vi "输入数据解析.vi"(0 "单个参数补充":dbl, 1 "从板号":dbl=1.0, 2 "主板二维码":string="BNET01", 3 "从板二维码":string="BNET01", 5 "主板引用":refnum<vi>, 7 "从板引用":refnum<vi>, 9 "主板选项":string="三级故障阀值", 11 "枚举":enum16{"主板", "从板"}(ring), 12 "快换":bool caption="快换写入") -> (4 "输出数组":dbl[][](array[numeric]), 6 "数组长度":dbl[](array[numeric]), 8 "循环次数":i32, 10 "命令":u32, 14 "名称":string[](array[string]), 15 "命令序号":u32[](array[numeric]))   [LabVIEW 2013] (continued)
                  }
                  frame Enabled {
                    w11585 = 255 ("高字节1")
                  }
                }
                n4442 = Build Array(w11577, w11578) -> (w11576:i32[])
              }
              frame 2 {
                # "温度过高"
                n4443 = disable-structure shown="启用" {
                  disable-tunnel: [w11592 255 ("高字节1")] -> w11588
                  disable-tunnel: w11586 -> [w11590 _]
                  frame Disabled {
                    n4444 = Unbundle By Name(w11590) -> ("温度过高"=w11589:dbl)
                    n4445 = call "输入分辨率计算-EV05.vi"("1字节?"=TRUE, "数值"=w11589, "偏移量"=-40.0, "分辨率"=1.0) -> ("高字节1"=w11592:dbl)  [unwired: 1 in, 6 out]
                  }
                  frame Enabled {
                  }
                }
                n4446 = Build Array(w11588) -> (w11587:i32[])
              }
              frame 3 {
                # "温度过低"
                n4447 = disable-structure shown="启用" {
                  disable-tunnel: [w11602 255 ("高字节1")] -> w11598
                  disable-tunnel: w11596 -> [w11600 _]
                  frame Disabled {
                    n4448 = Unbundle By Name(w11600) -> ("温度过低"=w11599:dbl)
                    n4449 = call "输入分辨率计算-EV05.vi"("1字节?"=TRUE, "数值"=w11599, "偏移量"=-40.0, "分辨率"=1.0) -> ("高字节1"=w11602:dbl)  [unwired: 1 in, 6 out]
                  }
                  frame Enabled {
                  }
                }
                n4450 = Build Array(w11598) -> (w11597:i32[])
              }
              frame 4 {
                # "整组温度不均衡"
                n4451 = disable-structure shown="启用" {
                  disable-tunnel: [w11612 255 ("高字节1")] -> w11608
                  disable-tunnel: w11606 -> [w11610 _]
                  frame Disabled {
                    n4452 = Unbundle By Name(w11610) -> ("整组温度不均衡"=w11609:dbl)
                    n4453 = call "输入分辨率计算-EV05.vi"("1字节?"=TRUE, "数值"=w11609, "偏移量"=0.0, "分辨率"=1.0) -> ("高字节1"=w11612:dbl)  [unwired: 1 in, 6 out]
                  }
                  frame Enabled {
                  }
                }
                n4454 = Build Array(w11608) -> (w11607:i32[])
              }
              frame 5 {
                # "单组电压不均衡"
                n4455 = disable-structure shown="启用" {
                  disable-tunnel: [w11624 w11627] -> w11619
                  disable-tunnel: [w11622 w11627] -> w11617
                  disable-tunnel: w11616 -> [w11621 _]
                  frame Disabled {
                    n4456 = Unbundle By Name(w11621) -> ("单组电压不均衡"=w11620:dbl)
                    n4457 = call "输入分辨率计算-EV05.vi"("1字节?"=FALSE, "数值"=w11620, "偏移量"=0.0, "分辨率"=0.001) -> ("低字节"=w11622:dbl, "高字节1"=w11624:dbl)  [unwired: 1 in, 5 out]
                  }
                  frame Enabled {
                    w11627 = 255 ("高字节1")
                  }
                }
                n4458 = Build Array(w11619, w11617) -> (w11618:i32[])
              }
              frame 6 {
                # "整组电压不均衡"
                n4459 = disable-structure shown="启用" {
                  disable-tunnel: [w11636 w11639] -> w11631
                  disable-tunnel: [w11634 w11639] -> w11629
                  disable-tunnel: w11628 -> [w11633 _]
                  frame Disabled {
                    n4460 = Unbundle By Name(w11633) -> ("整组电压不均衡"=w11632:dbl)
                    n4461 = call "输入分辨率计算-EV05.vi"("1字节?"=FALSE, "数值"=w11632, "偏移量"=0.0, "分辨率"=0.001) -> ("低字节"=w11634:dbl, "高字节1"=w11636:dbl)  [unwired: 1 in, 5 out]
                  }
                  frame Enabled {
                    w11639 = 255 ("高字节1")
                  }
                }
                n4462 = Build Array(w11631, w11629) -> (w11630:i32[])
              }
              frame 7 {
                # "单体电压过高"
                n4463 = disable-structure shown="启用" {
                  disable-tunnel: [w11648 w11651] -> w11643
                  disable-tunnel: [w11646 w11651] -> w11641
                  disable-tunnel: w11640 -> [w11645 _]
                  frame Disabled {
                    n4464 = Unbundle By Name(w11645) -> ("单体电压过高"=w11644:dbl)
                    n4465 = call "输入分辨率计算-EV05.vi"("1字节?"=FALSE, "数值"=w11644, "偏移量"=0.0, "分辨率"=0.001) -> ("低字节"=w11646:dbl, "高字节1"=w11648:dbl)  [unwired: 1 in, 5 out]
                  }
                  frame Enabled {
                    w11651 = 255 ("高字节1")
                  }
                }
                n4466 = Build Array(w11643, w11641) -> (w11642:i32[])
              }
              frame 8 {
                # "单体电压过低"
                n4467 = disable-structure shown="启用" {
                  disable-tunnel: [w11660 w11663] -> w11655
                  disable-tunnel: [w11658 w11663] -> w11653
                  disable-tunnel: w11652 -> [w11657 _]
                  frame Disabled {
                    n4468 = Unbundle By Name(w11657) -> ("单体电压过低"=w11656:dbl)
                    n4469 = call "输入分辨率计算-EV05.vi"("1字节?"=FALSE, "数值"=w11656, "偏移量"=0.0, "分辨率"=0.001) -> ("低字节"=w11658:dbl, "高字节1"=w11660:dbl)  [unwired: 1 in, 5 out]
                  }
                  frame Enabled {
                    w11663 = 255 ("高字节1")
                  }
                }
                n4470 = Build Array(w11655, w11653) -> (w11654:i32[])
              }
              frame 9 {
                # "充电电流过高"
                n4471 = disable-structure shown="启用" {
                  disable-tunnel: [w11672 w11675] -> w11667
                  disable-tunnel: [w11670 w11675] -> w11665
                  disable-tunnel: w11664 -> [w11669 _]
                  frame Disabled {
                    n4472 = Unbundle By Name(w11669) -> ("充电电流过高"=w11668:dbl)
                    n4473 = call "输入分辨率计算-EV05.vi"("1字节?"=FALSE, "数值"=w11668, "偏移量"=-3000.0, "分辨率"=0.1) -> ("低字节"=w11670:dbl, "高字节1"=w11672:dbl)  [unwired: 1 in, 5 out]
                  }
                  frame Enabled {
                    w11675 = 255 ("高字节1")
                  }
                }
                n4474 = Build Array(w11667, w11665) -> (w11666:i32[])
              }
              frame 10 {
                # "放电电流过高"
                n4475 = disable-structure shown="启用" {
                  disable-tunnel: [w11684 w11687] -> w11679
                  disable-tunnel: [w11682 w11687] -> w11677
                  disable-tunnel: w11676 -> [w11681 _]
                  frame Disabled {
                    n4476 = Unbundle By Name(w11681) -> ("放电电流过高"=w11680:dbl)
                    n4477 = call "输入分辨率计算-EV05.vi"("1字节?"=FALSE, "数值"=w11680, "偏移量"=-3000.0, "分辨率"=0.1) -> ("低字节"=w11682:dbl, "高字节1"=w11684:dbl)  [unwired: 1 in, 5 out]
                  }
                  frame Enabled {
                    w11687 = 255 ("高字节1")
                  }
                }
                n4478 = Build Array(w11679, w11677) -> (w11678:i32[])
              }
              frame 11 {
                # "单组温度不均衡"
                n4479 = disable-structure shown="启用" {
                  disable-tunnel: [w11694 255 ("高字节1")] -> w11690
                  disable-tunnel: w11688 -> [w11692 _]
                  frame Disabled {
                    n4480 = Unbundle By Name(w11692) -> ("单组温度不均衡"=w11691:dbl)
                    n4481 = call "输入分辨率计算-EV05.vi"("1字节?"=TRUE, "数值"=w11691, "偏移量"=0.0, "分辨率"=1.0) -> ("高字节1"=w11694:dbl)  [unwired: 1 in, 6 out]
                  }
                  frame Enabled {
                  }
                }
                n4482 = Build Array(w11690) -> (w11689:i32[])
              }
              frame 12 {
                # "SOC过高"
                n4483 = Unbundle By Name(w11701) -> ("SOC过高"=w11700:dbl)
                n4484 = call "输入分辨率计算-EV05.vi"("1字节?"=FALSE, "数值"=w11700, "偏移量"=0.0, "分辨率"=0.1) -> ("低字节"=w11698:dbl, "高字节1"=w11699:dbl)  [unwired: 1 in, 5 out]
                n4485 = Build Array(w11699, w11698) -> (w11703:dbl[])
              }
              frame 13 {
                # "SOC过低"
                n4486 = disable-structure shown="启用" {
                  disable-tunnel: w11708 -> [w11713 _]
                  disable-tunnel: [w11711 w11717] -> w11707
                  disable-tunnel: [w11710 w11717] -> w11706
                  frame Disabled {
                    n4487 = Unbundle By Name(w11713) -> ("SOC过低"=w11712:dbl)
                    n4488 = call "输入分辨率计算-EV05.vi"("1字节?"=FALSE, "数值"=w11712, "偏移量"=0.0, "分辨率"=0.1) -> ("低字节"=w11710:dbl, "高字节1"=w11711:dbl)  [unwired: 1 in, 5 out]
                  }
                  frame Enabled {
                    w11717 = 255 ("高字节1")
                  }
                }
                n4489 = Build Array(w11707, w11706) -> (w11709:i32[])
              }
              frame 14 {
                # "内阻过大"
                n4490 = disable-structure shown="启用" {
                  disable-tunnel: w11720 -> [w11725 _]
                  disable-tunnel: [w11721 255 ("高字节1")] -> w11718
                  frame Disabled {
                    n4491 = Unbundle By Name(w11725) -> ("内阻过大"=w11724:dbl)
                    n4492 = call "输入分辨率计算-EV05.vi"("1字节?"=TRUE, "数值"=w11724, "分辨率"=0.1) -> ("高字节1"=w11721:dbl)  [unwired: 2 in, 6 out]
                  }
                  frame Enabled {
                  }
                }
                n4493 = Build Array(w11718) -> (w11719:i32[])
              }
              frame 15 {
                # "极柱温度过高"
                n4494 = disable-structure shown="启用" {
                  disable-tunnel: w11729 -> [w11735 _]
                  disable-tunnel: [w11731 255 ("高字节1")] -> w11727
                  frame Disabled {
                    n4495 = Unbundle By Name(w11735) -> ("极柱温度过高"=w11734:dbl)
                    n4496 = call "输入分辨率计算-EV05.vi"("1字节?"=TRUE, "数值"=w11734, "偏移量"=-40.0, "分辨率"=1.0) -> ("高字节1"=w11731:dbl)  [unwired: 1 in, 6 out]
                  }
                  frame Enabled {
                  }
                }
                n4497 = Build Array(w11727) -> (w11728:i32[])
              }
              frame 16 {
                # "SOH过低"
                n4498 = disable-structure shown="启用" {
                  disable-tunnel: [w11752 w11760] -> w11739
                  disable-tunnel: w11738 -> [w11749 _]
                  disable-tunnel: [w11741 w11760] -> w11737
                  frame Disabled {
                    n4499 = Unbundle By Name(w11749) -> ("SOH过低"=w11748:dbl)
                    n4500 = call "输入分辨率计算-EV05.vi"("1字节?"=FALSE, "数值"=w11748, "偏移量"=0.0, "分辨率"=0.1) -> ("低字节"=w11750:dbl, "高字节1"=w11751:dbl)  [unwired: 1 in, 5 out]
                    n4501 = call "二进制解析-8.6.vi"("索引"=4, "数值"=w11751) -> ("低位子数组"=w11754:i32[])  [unwired: 3 out]
                    n4502 = call "二进制解析-8.6.vi"("索引"=4, "数值"=w11750) -> ("低位子数组"=w11743:i32[], "高位子数组"=w11753:i32[])  [unwired: 2 out]
                    n4503 = call "二进制解析-8.6.vi"("索引"=4, "数值"=0) -> ("低位子数组"=w11744:i32[])  [unwired: 3 out]
                    n4504 = Insert Into Array(array=w11754, new element=w11753) -> (w11747:i32[])  [unwired: 1 in]
                    n4505 = Insert Into Array(array=w11743, new element=w11744) -> (w11742:i32[])  [unwired: 1 in]
                    n4506 = call "数值二进制转十进制-8.6.vi"("子数组"=w11747) -> ("十进制数值"=w11752:i32)  [unwired: 4 out]
                    n4507 = call "数值二进制转十进制-8.6.vi"("子数组"=w11742) -> ("十进制数值"=w11741:i32)  [unwired: 4 out]
                  }
                  frame Enabled {
                    w11760 = 255 ("高字节1")
                  }
                }
                n4508 = Build Array(w11739, w11737) -> (w11740:i32[])
              }
            }
            n4509 = Insert Into Array(array=w11560, new element=w11561) -> (w11559:dbl[])  [unwired: 1 in]
          }
          n4510 = Build Array(w11556) -> (w11555:dbl[][])
          n4511 = Build Array("二级故障阀值") -> (w11546:string[])
        }
        frame "SOC过高(3)" {
          n4512 = Unbundle By Name(w11766) -> ("一级故障 3"=w11767:refnum<vi>)
          n4513 = property class="Clust (严格)"(reference=w11767) -> ("Value"=w11765:T4)  [unwired: 1 in, 2 out]
          n4514 = for {
            N: 17 -> [_]
            tunnel: w11765 -> [w11777]
            shift-right: [w11774] -> w11771
            shift-left: dbl[] [] -> [w11775]
            i -> [w11778]
            n4515 = case shown="12" w11778 {
              tunnel: w11777 -> [w11779 w11790 w11801 w11811 w11821 w11831 w11843 w11855 w11867 w11879 w11891 w11903 w11916 w11924 w11931 w11940 w11949]
              tunnel: [w11780 w11791 w11802 w11812 w11822 w11833 w11845 w11857 w11869 w11881 w11893 w11904 w11918 w11926 w11930 w11939 w11951] -> w11776
              frame 0, Default {
                # "总电压过高"
                n4516 = disable-structure shown="启用" {
                  disable-tunnel: [w11786 w11789] -> w11782
                  disable-tunnel: [w11785 w11789] -> w11781
                  disable-tunnel: w11779 -> [w11784 _]
                  frame Disabled {
                    n4517 = Unbundle By Name(w11784) -> ("总电压过高"=w11783:dbl)
                    n4518 = call "输入分辨率计算-EV05.vi"("1字节?"=FALSE, "数值"=w11783, "分辨率"=0.1) -> ("低字节"=w11786:dbl, "高字节1"=w11785:dbl)  [unwired: 2 in, 5 out]
                  }
                  frame Enabled {
                    w11789 = 255 ("高字节1")
                  }
                }
                n4519 = Build Array(w11781, w11782) -> (w11780:i32[])
              }
              frame 1 {
                # "总电压过低"
                n4520 = disable-structure shown="启用" {
                  disable-tunnel: [w11797 w11800] -> w11793
                  disable-tunnel: [w11796 w11800] -> w11792
                  disable-tunnel: w11790 -> [w11795 _]
                  frame Disabled {
                    n4521 = Unbundle By Name(w11795) -> ("总电压过低"=w11794:dbl)
                    n4522 = call "输入分辨率计算-EV05.vi"("1字节?"=FALSE, "数值"=w11794, "分辨率"=0.1) -> ("低字节"=w11797:dbl, "高字节1"=w11796:dbl)  [unwired: 2 in, 5 out]
                  }
                  frame Enabled {
                    w11800 = 255 ("高字节1")
                  }
                }
                n4523 = Build Array(w11792, w11793) -> (w11791:i32[])
              }
              frame 2 {
                # "温度过高"
                n4524 = disable-structure shown="启用" {
                  disable-tunnel: [w11807 255 ("高字节1")] -> w11803
                  disable-tunnel: w11801 -> [w11805 _]
                  frame Disabled {
                    n4525 = Unbundle By Name(w11805) -> ("温度过高"=w11804:dbl)
                    n4526 = call "输入分辨率计算-EV05.vi"("1字节?"=TRUE, "数值"=w11804, "偏移量"=-40.0, "分辨率"=1.0) -> ("高字节1"=w11807:dbl)  [unwired: 1 in, 6 out]
                  }
                  frame Enabled {
                  }
                }
                n4527 = Build Array(w11803) -> (w11802:i32[])
              }
              frame 3 {
                # "温度过低"
                n4528 = disable-structure shown="启用" {
                  disable-tunnel: [w11817 255 ("高字节1")] -> w11813
                  disable-tunnel: w11811 -> [w11815 _]
                  frame Disabled {
                    n4529 = Unbundle By Name(w11815) -> ("温度过低"=w11814:dbl)
                    n4530 = call "输入分辨率计算-EV05.vi"("1字节?"=TRUE, "数值"=w11814, "偏移量"=-40.0, "分辨率"=1.0) -> ("高字节1"=w11817:dbl)  [unwired: 1 in, 6 out]
                  }
                  frame Enabled {
                  }
                }
                n4531 = Build Array(w11813) -> (w11812:i32[])
              }
              frame 4 {
                # "整组温度不均衡"
                n4532 = disable-structure shown="启用" {
                  disable-tunnel: [w11827 255 ("高字节1")] -> w11823
                  disable-tunnel: w11821 -> [w11825 _]
                  frame Disabled {
                    n4533 = Unbundle By Name(w11825) -> ("整组温度不均衡"=w11824:dbl)
                    n4534 = call "输入分辨率计算-EV05.vi"("1字节?"=TRUE, "数值"=w11824, "偏移量"=0.0, "分辨率"=1.0) -> ("高字节1"=w11827:dbl)  [unwired: 1 in, 6 out]
                  }
                  frame Enabled {
                  }
                }
                n4535 = Build Array(w11823) -> (w11822:i32[])
              }
              frame 5 {
                # "单组电压不均衡"
                n4536 = disable-structure shown="启用" {
                  disable-tunnel: [w11839 w11842] -> w11834
                  disable-tunnel: [w11837 w11842] -> w11832
                  disable-tunnel: w11831 -> [w11836 _]
                  frame Disabled {
                    n4537 = Unbundle By Name(w11836) -> ("单组电压不均衡"=w11835:dbl)
                    n4538 = call "输入分辨率计算-EV05.vi"("1字节?"=FALSE, "数值"=w11835, "偏移量"=0.0, "分辨率"=0.001) -> ("低字节"=w11837:dbl, "高字节1"=w11839:dbl)  [unwired: 1 in, 5 out]
                  }
                  frame Enabled {
                    w11842 = 255 ("高字节1")
                  }
                }
                n4539 = Build Array(w11834, w11832) -> (w11833:i32[])
              }
              frame 6 {
                # "整组电压不均衡"
                n4540 = disable-structure shown="启用" {
                  disable-tunnel: [w11851 w11854] -> w11846
                  disable-tunnel: [w11849 w11854] -> w11844
                  disable-tunnel: w11843 -> [w11848 _]
                  frame Disabled {
                    n4541 = Unbundle By Name(w11848) -> ("整组电压不均衡"=w11847:dbl)
                    n4542 = call "输入分辨率计算-EV05.vi"("1字节?"=FALSE, "数值"=w11847, "偏移量"=0.0, "分辨率"=0.001) -> ("低字节"=w11849:dbl, "高字节1"=w11851:dbl)  [unwired: 1 in, 5 out]
                  }
                  frame Enabled {
                    w11854 = 255 ("高字节1")
                  }
                }
                n4543 = Build Array(w11846, w11844) -> (w11845:i32[])
              }
              frame 7 {
                # "单体电压过高"
                n4544 = disable-structure shown="启用" {
                  disable-tunnel: [w11863 w11866] -> w11858
                  disable-tunnel: [w11861 w11866] -> w11856
                  disable-tunnel: w11855 -> [w11860 _]
                  frame Disabled {
                    n4545 = Unbundle By Name(w11860) -> ("单体电压过高"=w11859:dbl)
                    n4546 = call "输入分辨率计算-EV05.vi"("1字节?"=FALSE, "数值"=w11859, "偏移量"=0.0, "分辨率"=0.001) -> ("低字节"=w11861:dbl, "高字节1"=w11863:dbl)  [unwired: 1 in, 5 out]
                  }
                  frame Enabled {
                    w11866 = 255 ("高字节1")
                  }
                }
                n4547 = Build Array(w11858, w11856) -> (w11857:i32[])
              }
              frame 8 {
                # "单体电压过低"
                n4548 = disable-structure shown="启用" {
                  disable-tunnel: [w11875 w11878] -> w11870
                  disable-tunnel: [w11873 w11878] -> w11868
                  disable-tunnel: w11867 -> [w11872 _]
                  frame Disabled {
                    n4549 = Unbundle By Name(w11872) -> ("单体电压过低"=w11871:dbl)
                    n4550 = call "输入分辨率计算-EV05.vi"("1字节?"=FALSE, "数值"=w11871, "偏移量"=0.0, "分辨率"=0.001) -> ("低字节"=w11873:dbl, "高字节1"=w11875:dbl)  [unwired: 1 in, 5 out]
                  }
                  frame Enabled {
                    w11878 = 255 ("高字节1")
                  }
                }
                n4551 = Build Array(w11870, w11868) -> (w11869:i32[])
              }
              frame 9 {
                # "充电电流过高"
                n4552 = disable-structure shown="启用" {
                  disable-tunnel: [w11887 w11890] -> w11882
                  disable-tunnel: [w11885 w11890] -> w11880
                  disable-tunnel: w11879 -> [w11884 _]
                  frame Disabled {
                    n4553 = Unbundle By Name(w11884) -> ("充电电流过高"=w11883:dbl)
                    n4554 = call "输入分辨率计算-EV05.vi"("1字节?"=FALSE, "数值"=w11883, "偏移量"=-3000.0, "分辨率"=0.1) -> ("低字节"=w11885:dbl, "高字节1"=w11887:dbl)  [unwired: 1 in, 5 out]
                  }
                  frame Enabled {
                    w11890 = 255 ("高字节1")
                  }
                }
                n4555 = Build Array(w11882, w11880) -> (w11881:i32[])
              }
              frame 10 {
                # "放电电流过高"
                n4556 = disable-structure shown="启用" {
                  disable-tunnel: [w11899 w11902] -> w11894
                  disable-tunnel: [w11897 w11902] -> w11892
                  disable-tunnel: w11891 -> [w11896 _]
                  frame Disabled {
                    n4557 = Unbundle By Name(w11896) -> ("放电电流过高"=w11895:dbl)
                    n4558 = call "输入分辨率计算-EV05.vi"("1字节?"=FALSE, "数值"=w11895, "偏移量"=-3000.0, "分辨率"=0.1) -> ("低字节"=w11897:dbl, "高字节1"=w11899:dbl)  [unwired: 1 in, 5 out]
                  }
                  frame Enabled {
                    w11902 = 255 ("高字节1")
                  }
                }
                n4559 = Build Array(w11894, w11892) -> (w11893:i32[])
              }
              frame 11 {
                # "单组温度不均衡"
                n4560 = disable-structure shown="启用" {
                  disable-tunnel: [w11909 255 ("高字节1")] -> w11905
                  disable-tunnel: w11903 -> [w11907 _]
                  frame Disabled {
                    n4561 = Unbundle By Name(w11907) -> ("单组温度不均衡"=w11906:dbl)
                    n4562 = call "输入分辨率计算-EV05.vi"("1字节?"=TRUE, "数值"=w11906, "偏移量"=0.0, "分辨率"=1.0) -> ("高字节1"=w11909:dbl)  [unwired: 1 in, 6 out]
                  }
                  frame Enabled {
                  }
                }
                n4563 = Build Array(w11905) -> (w11904:i32[])
              }
              frame 12 {
                # "SOC过高"
                n4564 = Unbundle By Name(w11916) -> ("SOC过高"=w11915:dbl)
                n4565 = call "输入分辨率计算-EV05.vi"("1字节?"=FALSE, "数值"=w11915, "偏移量"=0.0, "分辨率"=0.1) -> ("低字节"=w11913:dbl, "高字节1"=w11914:dbl)  [unwired: 1 in, 5 out]
                n4566 = Build Array(w11914, w11913) -> (w11918:dbl[])
              }
              frame 13 {
                # "SOC过低"
                n4567 = Unbundle By Name(w11924) -> ("SOC过低"=w11923:dbl)
                n4568 = call "输入分辨率计算-EV05.vi"("1字节?"=FALSE, "数值"=w11923, "偏移量"=0.0, "分辨率"=0.1) -> ("低字节"=w11921:dbl, "高字节1"=w11922:dbl)  [unwired: 1 in, 5 out]
                n4569 = Build Array(w11922, w11921) -> (w11926:dbl[])
              }
              frame 14 {
                # "内阻过大"
                n4570 = disable-structure shown="启用" {
                  disable-tunnel: w11931 -> [w11936 _]
                  disable-tunnel: [w11932 255 ("高字节1")] -> w11929
                  frame Disabled {
                    n4571 = Unbundle By Name(w11936) -> ("内阻过大"=w11935:dbl)
                    n4572 = call "输入分辨率计算-EV05.vi"("1字节?"=TRUE, "数值"=w11935, "分辨率"=0.1) -> ("高字节1"=w11932:dbl)  [unwired: 2 in, 6 out]
                  }
                  frame Enabled {
                  }
                }
                n4573 = Build Array(w11929) -> (w11930:i32[])
              }
              frame 15 {
                # "极柱温度过高"
                n4574 = disable-structure shown="启用" {
                  disable-tunnel: w11940 -> [w11946 _]
                  disable-tunnel: [w11942 255 ("高字节1")] -> w11938
                  frame Disabled {
                    n4575 = Unbundle By Name(w11946) -> ("极柱温度过高"=w11945:dbl)
                    n4576 = call "输入分辨率计算-EV05.vi"("1字节?"=TRUE, "数值"=w11945, "偏移量"=-40.0, "分辨率"=1.0) -> ("高字节1"=w11942:dbl)  [unwired: 1 in, 6 out]
                  }
                  frame Enabled {
                  }
                }
                n4577 = Build Array(w11938) -> (w11939:i32[])
              }
              frame 16 {
                # "SOH过低"
                n4578 = disable-structure shown="启用" {
                  disable-tunnel: [w11963 w11971] -> w11950
                  disable-tunnel: w11949 -> [w11960 _]
                  disable-tunnel: [w11952 w11971] -> w11948
                  frame Disabled {
                    n4579 = Unbundle By Name(w11960) -> ("SOH过低"=w11959:dbl)
                    n4580 = call "输入分辨率计算-EV05.vi"("1字节?"=FALSE, "数值"=w11959, "偏移量"=0.0, "分辨率"=0.1) -> ("低字节"=w11961:dbl, "高字节1"=w11962:dbl)  [unwired: 1 in, 5 out]
                    n4581 = call "二进制解析-8.6.vi"("索引"=4, "数值"=w11962) -> ("低位子数组"=w11965:i32[])  [unwired: 3 out]
                    n4582 = call "二进制解析-8.6.vi"("索引"=4, "数值"=w11961) -> ("低位子数组"=w11954:i32[], "高位子数组"=w11964:i32[])  [unwired: 2 out]
                    n4583 = call "二进制解析-8.6.vi"("索引"=4, "数值"=0) -> ("低位子数组"=w11955:i32[])  [unwired: 3 out]
                    n4584 = Insert Into Array(array=w11965, new element=w11964) -> (w11958:i32[])  [unwired: 1 in]
                    n4585 = Insert Into Array(array=w11954, new element=w11955) -> (w11953:i32[])  [unwired: 1 in]
                    n4586 = call "数值二进制转十进制-8.6.vi"("子数组"=w11958) -> ("十进制数值"=w11963:i32)  [unwired: 4 out]
                    n4587 = call "数值二进制转十进制-8.6.vi"("子数组"=w11953) -> ("十进制数值"=w11952:i32)  [unwired: 4 out]
                  }
                  frame Enabled {
                    w11971 = 255 ("高字节1")
                  }
                }
                n4588 = Build Array(w11950, w11948) -> (w11951:i32[])
              }
            }
            n4589 = Insert Into Array(array=w11775, new element=w11776) -> (w11774:dbl[])  [unwired: 1 in]
          }
          n4590 = Build Array(w11771) -> (w11770:dbl[][])
          n4591 = Build Array("三级故障阀值") -> (w11761:string[])
        }
        frame "SOC过低" {
          n4592 = Unbundle By Name(w11977) -> ("一级故障"=w11978:refnum<vi>)
          n4593 = property class="Clust (严格)"(reference=w11978) -> ("Value"=w11976:T4)  [unwired: 1 in, 2 out]
          n4594 = for {
            N: 17 -> [_]
            tunnel: w11976 -> [w11988]
            shift-right: [w11985] -> w11982
            shift-left: dbl[] [] -> [w11986]
            i -> [w11989]
            n4595 = case shown="12" w11989 {
              tunnel: w11988 -> [w11990 w12001 w12012 w12022 w12032 w12042 w12054 w12066 w12078 w12090 w12102 w12114 w12126 w12138 w12145 w12154 w12163]
              tunnel: [w11991 w12002 w12013 w12023 w12033 w12044 w12056 w12068 w12080 w12092 w12104 w12115 w12128 w12140 w12144 w12153 w12165] -> w11987
              frame 0, Default {
                # "总电压过高"
                n4596 = disable-structure shown="启用" {
                  disable-tunnel: [w11997 w12000] -> w11993
                  disable-tunnel: [w11996 w12000] -> w11992
                  disable-tunnel: w11990 -> [w11995 _]
                  frame Disabled {
                    n4597 = Unbundle By Name(w11995) -> ("总电压过高"=w11994:dbl)
                    n4598 = call "输入分辨率计算-EV05.vi"("1字节?"=FALSE, "数值"=w11994, "分辨率"=0.1) -> ("低字节"=w11997:dbl, "高字节1"=w11996:dbl)  [unwired: 2 in, 5 out]
                  }
                  frame Enabled {
                    w12000 = 255 ("高字节1")
                  }
                }
                n4599 = Build Array(w11992, w11993) -> (w11991:i32[])
              }
              frame 1 {
                # "总电压过低"
                n4600 = disable-structure shown="启用" {
                  disable-tunnel: [w12008 w12011] -> w12004
                  disable-tunnel: [w12007 w12011] -> w12003
                  disable-tunnel: w12001 -> [w12006 _]
                  frame Disabled {
                    n4601 = Unbundle By Name(w12006) -> ("总电压过低"=w12005:dbl)
                    n4602 = call "输入分辨率计算-EV05.vi"("1字节?"=FALSE, "数值"=w12005, "分辨率"=0.1) -> ("低字节"=w12008:dbl, "高字节1"=w12007:dbl)  [unwired: 2 in, 5 out]
                  }
                  frame Enabled {
                    w12011 = 255 ("高字节1")
                  }
                }
                n4603 = Build Array(w12003, w12004) -> (w12002:i32[])
              }
              frame 2 {
                # "温度过高"
                n4604 = disable-structure shown="启用" {
                  disable-tunnel: [w12018 255 ("高字节1")] -> w12014
                  disable-tunnel: w12012 -> [w12016 _]
                  frame Disabled {
                    n4605 = Unbundle By Name(w12016) -> ("温度过高"=w12015:dbl)
                    n4606 = call "输入分辨率计算-EV05.vi"("1字节?"=TRUE, "数值"=w12015, "偏移量"=-40.0, "分辨率"=1.0) -> ("高字节1"=w12018:dbl)  [unwired: 1 in, 6 out]
                  }
                  frame Enabled {
                  }
                }
                n4607 = Build Array(w12014) -> (w12013:i32[])
              }
              frame 3 {
                # "温度过低"
                n4608 = disable-structure shown="启用" {
                  disable-tunnel: [w12028 255 ("高字节1")] -> w12024
                  disable-tunnel: w12022 -> [w12026 _]
                  frame Disabled {
                    n4609 = Unbundle By Name(w12026) -> ("温度过低"=w12025:dbl)
                    n4610 = call "输入分辨率计算-EV05.vi"("1字节?"=TRUE, "数值"=w12025, "偏移量"=-40.0, "分辨率"=1.0) -> ("高字节1"=w12028:dbl)  [unwired: 1 in, 6 out]
                  }
                  frame Enabled {
                  }
                }
                n4611 = Build Array(w12024) -> (w12023:i32[])
              }
              frame 4 {
                # "整组温度不均衡"
                n4612 = disable-structure shown="启用" {
                  disable-tunnel: [w12038 255 ("高字节1")] -> w12034
                  disable-tunnel: w12032 -> [w12036 _]
                  frame Disabled {
                    n4613 = Unbundle By Name(w12036) -> ("整组温度不均衡"=w12035:dbl)
                    n4614 = call "输入分辨率计算-EV05.vi"("1字节?"=TRUE, "数值"=w12035, "偏移量"=0.0, "分辨率"=1.0) -> ("高字节1"=w12038:dbl)  [unwired: 1 in, 6 out]
                  }
                  frame Enabled {
                  }
                }
                n4615 = Build Array(w12034) -> (w12033:i32[])
              }
              frame 5 {
                # "单组电压不均衡"
                n4616 = disable-structure shown="启用" {
                  disable-tunnel: [w12050 w12053] -> w12045
                  disable-tunnel: [w12048 w12053] -> w12043
                  disable-tunnel: w12042 -> [w12047 _]
                  frame Disabled {
                    n4617 = Unbundle By Name(w12047) -> ("单组电压不均衡"=w12046:dbl)
                    n4618 = call "输入分辨率计算-EV05.vi"("1字节?"=FALSE, "数值"=w12046, "偏移量"=0.0, "分辨率"=0.001) -> ("低字节"=w12048:dbl, "高字节1"=w12050:dbl)  [unwired: 1 in, 5 out]
                  }
                  frame Enabled {
                    w12053 = 255 ("高字节1")
                  }
                }
                n4619 = Build Array(w12045, w12043) -> (w12044:i32[])
              }
              frame 6 {
                # "整组电压不均衡"
                n4620 = disable-structure shown="启用" {
                  disable-tunnel: [w12062 w12065] -> w12057
                  disable-tunnel: [w12060 w12065] -> w12055
                  disable-tunnel: w12054 -> [w12059 _]
                  frame Disabled {
                    n4621 = Unbundle By Name(w12059) -> ("整组电压不均衡"=w12058:dbl)
                    n4622 = call "输入分辨率计算-EV05.vi"("1字节?"=FALSE, "数值"=w12058, "偏移量"=0.0, "分辨率"=0.001) -> ("低字节"=w12060:dbl, "高字节1"=w12062:dbl)  [unwired: 1 in, 5 out]
                  }
                  frame Enabled {
                    w12065 = 255 ("高字节1")
                  }
                }
                n4623 = Build Array(w12057, w12055) -> (w12056:i32[])
              }
              frame 7 {
                # "单体电压过高"
                n4624 = disable-structure shown="启用" {
                  disable-tunnel: [w12074 w12077] -> w12069
                  disable-tunnel: [w12072 w12077] -> w12067
                  disable-tunnel: w12066 -> [w12071 _]
                  frame Disabled {
                    n4625 = Unbundle By Name(w12071) -> ("单体电压过高"=w12070:dbl)
                    n4626 = call "输入分辨率计算-EV05.vi"("1字节?"=FALSE, "数值"=w12070, "偏移量"=0.0, "分辨率"=0.001) -> ("低字节"=w12072:dbl, "高字节1"=w12074:dbl)  [unwired: 1 in, 5 out]
                  }
                  frame Enabled {
                    w12077 = 255 ("高字节1")
                  }
                }
                n4627 = Build Array(w12069, w12067) -> (w12068:i32[])
              }
              frame 8 {
                # "单体电压过低"
                n4628 = disable-structure shown="启用" {
                  disable-tunnel: [w12086 w12089] -> w12081
                  disable-tunnel: [w12084 w12089] -> w12079
                  disable-tunnel: w12078 -> [w12083 _]
                  frame Disabled {
                    n4629 = Unbundle By Name(w12083) -> ("单体电压过低"=w12082:dbl)
                    n4630 = call "输入分辨率计算-EV05.vi"("1字节?"=FALSE, "数值"=w12082, "偏移量"=0.0, "分辨率"=0.001) -> ("低字节"=w12084:dbl, "高字节1"=w12086:dbl)  [unwired: 1 in, 5 out]
                  }
                  frame Enabled {
                    w12089 = 255 ("高字节1")
                  }
                }
                n4631 = Build Array(w12081, w12079) -> (w12080:i32[])
              }
              frame 9 {
                # "充电电流过高"
                n4632 = disable-structure shown="启用" {
                  disable-tunnel: [w12098 w12101] -> w12093
                  disable-tunnel: [w12096 w12101] -> w12091
                  disable-tunnel: w12090 -> [w12095 _]
                  frame Disabled {
                    n4633 = Unbundle By Name(w12095) -> ("充电电流过高"=w12094:dbl)
                    n4634 = call "输入分辨率计算-EV05.vi"("1字节?"=FALSE, "数值"=w12094, "偏移量"=-3000.0, "分辨率"=0.1) -> ("低字节"=w12096:dbl, "高字节1"=w12098:dbl)  [unwired: 1 in, 5 out]
                  }
                  frame Enabled {
                    w12101 = 255 ("高字节1")
                  }
                }
                n4635 = Build Array(w12093, w12091) -> (w12092:i32[])
              }
              frame 10 {
                # "放电电流过高"
                n4636 = disable-structure shown="启用" {
                  disable-tunnel: [w12110 w12113] -> w12105
                  disable-tunnel: [w12108 w12113] -> w12103
                  disable-tunnel: w12102 -> [w12107 _]
                  frame Disabled {
                    n4637 = Unbundle By Name(w12107) -> ("放电电流过高"=w12106:dbl)
                    n4638 = call "输入分辨率计算-EV05.vi"("1字节?"=FALSE, "数值"=w12106, "偏移量"=-3000.0, "分辨率"=0.1) -> ("低字节"=w12108:dbl, "高字节1"=w12110:dbl)  [unwired: 1 in, 5 out]
                  }
                  frame Enabled {
                    w12113 = 255 ("高字节1")
                  }
                }
                n4639 = Build Array(w12105, w12103) -> (w12104:i32[])
              }
              frame 11 {
                # "单组温度不均衡"
                n4640 = disable-structure shown="启用" {
                  disable-tunnel: [w12120 255 ("高字节1")] -> w12116
                  disable-tunnel: w12114 -> [w12118 _]
                  frame Disabled {
                    n4641 = Unbundle By Name(w12118) -> ("单组温度不均衡"=w12117:dbl)
                    n4642 = call "输入分辨率计算-EV05.vi"("1字节?"=TRUE, "数值"=w12117, "偏移量"=0.0, "分辨率"=1.0) -> ("高字节1"=w12120:dbl)  [unwired: 1 in, 6 out]
                  }
                  frame Enabled {
                  }
                }
                n4643 = Build Array(w12116) -> (w12115:i32[])
              }
              frame 12 {
                # "SOC过高"
                n4644 = Unbundle By Name(w12126) -> ("SOC过高"=w12125:dbl)
                n4645 = call "输入分辨率计算-EV05.vi"("1字节?"=FALSE, "数值"=w12125, "偏移量"=0.0, "分辨率"=0.1) -> ()  [unwired: 1 in, 7 out]
                n4646 = disable-structure shown="启用" {
                  disable-tunnel: _ -> [w12132 _]
                  disable-tunnel: [w12132 255 ("高字节1")] -> w12124
                  disable-tunnel: [w12131 i32[] [] ("低位子数组")] -> _
                  disable-tunnel: _ -> [w12131 _]
                  frame Disabled {
                  }
                  frame Enabled {
                  }
                }
                n4647 = Build Array(w12124, w12124) -> (w12128:i32[])
              }
              frame 13 {
                # "SOC过低"
                n4648 = Unbundle By Name(w12138) -> ("SOC过低"=w12137:dbl)
                n4649 = call "输入分辨率计算-EV05.vi"("1字节?"=FALSE, "数值"=w12137, "偏移量"=0.0, "分辨率"=0.1) -> ("低字节"=w12135:dbl, "高字节1"=w12136:dbl)  [unwired: 1 in, 5 out]
                n4650 = Build Array(w12136, w12135) -> (w12140:dbl[])
              }
              frame 14 {
                # "内阻过大"
                n4651 = disable-structure shown="启用" {
                  disable-tunnel: w12145 -> [w12150 _]
                  disable-tunnel: [w12146 255 ("高字节1")] -> w12143
                  frame Disabled {
                    n4652 = Unbundle By Name(w12150) -> ("内阻过大"=w12149:dbl)
                    n4653 = call "输入分辨率计算-EV05.vi"("1字节?"=TRUE, "数值"=w12149, "分辨率"=0.1) -> ("高字节1"=w12146:dbl)  [unwired: 2 in, 6 out]
                  }
                  frame Enabled {
                  }
                }
                n4654 = Build Array(w12143) -> (w12144:i32[])
              }
              frame 15 {
                # "极柱温度过高"
                n4655 = disable-structure shown="启用" {
                  disable-tunnel: w12154 -> [w12160 _]
                  disable-tunnel: [w12156 255 ("高字节1")] -> w12152
                  frame Disabled {
                    n4656 = Unbundle By Name(w12160) -> ("极柱温度过高"=w12159:dbl)
                    n4657 = call "输入分辨率计算-EV05.vi"("1字节?"=TRUE, "数值"=w12159, "偏移量"=-40.0, "分辨率"=1.0) -> ("高字节1"=w12156:dbl)  [unwired: 1 in, 6 out]
                  }
                  frame Enabled {
                  }
                }
                n4658 = Build Array(w12152) -> (w12153:i32[])
              }
              frame 16 {
                # "SOH过低"
                n4659 = disable-structure shown="启用" {
                  disable-tunnel: [w12177 w12185] -> w12164
                  disable-tunnel: w12163 -> [w12174 _]
                  disable-tunnel: [w12166 w12185] -> w12162
                  frame Disabled {
                    n4660 = Unbundle By Name(w12174) -> ("SOH过低"=w12173:dbl)
                    n4661 = call "输入分辨率计算-EV05.vi"("1字节?"=FALSE, "数值"=w12173, "偏移量"=0.0, "分辨率"=0.1) -> ("低字节"=w12175:dbl, "高字节1"=w12176:dbl)  [unwired: 1 in, 5 out]
                    n4662 = call "二进制解析-8.6.vi"("索引"=4, "数值"=w12176) -> ("低位子数组"=w12179:i32[])  [unwired: 3 out]
                    n4663 = call "二进制解析-8.6.vi"("索引"=4, "数值"=w12175) -> ("低位子数组"=w12168:i32[], "高位子数组"=w12178:i32[])  [unwired: 2 out]
                    n4664 = call "二进制解析-8.6.vi"("索引"=4, "数值"=0) -> ("低位子数组"=w12169:i32[])  [unwired: 3 out]
                    n4665 = Insert Into Array(array=w12179, new element=w12178) -> (w12172:i32[])  [unwired: 1 in]
                    n4666 = Insert Into Array(array=w12168, new element=w12169) -> (w12167:i32[])  [unwired: 1 in]
                    n4667 = call "数值二进制转十进制-8.6.vi"("子数组"=w12172) -> ("十进制数值"=w12177:i32)  [unwired: 4 out]
                    n4668 = call "数值二进制转十进制-8.6.vi"("子数组"=w12167) -> ("十进制数值"=w12166:i32)  [unwired: 4 out]
                  }
                  frame Enabled {
                    w12185 = 255 ("高字节1")
                  }
                }
                n4669 = Build Array(w12164, w12162) -> (w12165:i32[])
              }
            }
            n4670 = Insert Into Array(array=w11986, new element=w11987) -> (w11985:dbl[])  [unwired: 1 in]
          }
          n4671 = Build Array(w11982) -> (w11981:dbl[][])
          n4672 = Build Array("一级故障阀值") -> (w11972:string[])
        }
        frame "SOC过低(2)" {
          n4673 = Unbundle By Name(w12191) -> ("一级故障 2"=w12192:refnum<vi>)
          n4674 = property class="Clust (严格)"(reference=w12192) -> ("Value"=w12190:T4)  [unwired: 1 in, 2 out]
          n4675 = for {
            N: 17 -> [_]
            tunnel: w12190 -> [w12202]
            shift-right: [w12199] -> w12196
            shift-left: dbl[] [] -> [w12200]
            i -> [w12203]
            n4676 = case shown="12" w12203 {
              tunnel: w12202 -> [w12204 w12215 w12226 w12236 w12246 w12256 w12268 w12280 w12292 w12304 w12316 w12328 w12340 w12352 w12359 w12368 w12377]
              tunnel: [w12205 w12216 w12227 w12237 w12247 w12258 w12270 w12282 w12294 w12306 w12318 w12329 w12342 w12354 w12358 w12367 w12379] -> w12201
              frame 0, Default {
                # "总电压过高"
                n4677 = disable-structure shown="启用" {
                  disable-tunnel: [w12211 w12214] -> w12207
                  disable-tunnel: [w12210 w12214] -> w12206
                  disable-tunnel: w12204 -> [w12209 _]
                  frame Disabled {
                    n4678 = Unbundle By Name(w12209) -> ("总电压过高"=w12208:dbl)
                    n4679 = call "输入分辨率计算-EV05.vi"("1字节?"=FALSE, "数值"=w12208, "分辨率"=0.1) -> ("低字节"=w12211:dbl, "高字节1"=w12210:dbl)  [unwired: 2 in, 5 out]
                  }
                  frame Enabled {
                    w12214 = 255 ("高字节1")
                  }
                }
                n4680 = Build Array(w12206, w12207) -> (w12205:i32[])
              }
              frame 1 {
                # "总电压过低"
                n4681 = disable-structure shown="启用" {
                  disable-tunnel: [w12222 w12225] -> w12218
                  disable-tunnel: [w12221 w12225] -> w12217
                  disable-tunnel: w12215 -> [w12220 _]
                  frame Disabled {
                    n4682 = Unbundle By Name(w12220) -> ("总电压过低"=w12219:dbl)
                    n4683 = call "输入分辨率计算-EV05.vi"("1字节?"=FALSE, "数值"=w12219, "分辨率"=0.1) -> ("低字节"=w12222:dbl, "高字节1"=w12221:dbl)  [unwired: 2 in, 5 out]
                  }
                  frame Enabled {
                    w12225 = 255 ("高字节1")
                  }
                }
                n4684 = Build Array(w12217, w12218) -> (w12216:i32[])
              }
              frame 2 {
                # "温度过高"
                n4685 = disable-structure shown="启用" {
                  disable-tunnel: [w12232 255 ("高字节1")] -> w12228
                  disable-tunnel: w12226 -> [w12230 _]
                  frame Disabled {
                    n4686 = Unbundle By Name(w12230) -> ("温度过高"=w12229:dbl)
                    n4687 = call "输入分辨率计算-EV05.vi"("1字节?"=TRUE, "数值"=w12229, "偏移量"=-40.0, "分辨率"=1.0) -> ("高字节1"=w12232:dbl)  [unwired: 1 in, 6 out]
                  }
                  frame Enabled {
                  }
                }
                n4688 = Build Array(w12228) -> (w12227:i32[])
              }
              frame 3 {
                # "温度过低"
                n4689 = disable-structure shown="启用" {
                  disable-tunnel: [w12242 255 ("高字节1")] -> w12238
                  disable-tunnel: w12236 -> [w12240 _]
                  frame Disabled {
                    n4690 = Unbundle By Name(w12240) -> ("温度过低"=w12239:dbl)
                    n4691 = call "输入分辨率计算-EV05.vi"("1字节?"=TRUE, "数值"=w12239, "偏移量"=-40.0, "分辨率"=1.0) -> ("高字节1"=w12242:dbl)  [unwired: 1 in, 6 out]
                  }
                  frame Enabled {
                  }
                }
                n4692 = Build Array(w12238) -> (w12237:i32[])
              }
              frame 4 {
                # "整组温度不均衡"
                n4693 = disable-structure shown="启用" {
                  disable-tunnel: [w12252 255 ("高字节1")] -> w12248
                  disable-tunnel: w12246 -> [w12250 _]
                  frame Disabled {
                    n4694 = Unbundle By Name(w12250) -> ("整组温度不均衡"=w12249:dbl)
                    n4695 = call "输入分辨率计算-EV05.vi"("1字节?"=TRUE, "数值"=w12249, "偏移量"=0.0, "分辨率"=1.0) -> ("高字节1"=w12252:dbl)  [unwired: 1 in, 6 out]
                  }
                  frame Enabled {
                  }
                }
                n4696 = Build Array(w12248) -> (w12247:i32[])
              }
              frame 5 {
                # "单组电压不均衡"
                n4697 = disable-structure shown="启用" {
                  disable-tunnel: [w12264 w12267] -> w12259
                  disable-tunnel: [w12262 w12267] -> w12257
                  disable-tunnel: w12256 -> [w12261 _]
                  frame Disabled {
                    n4698 = Unbundle By Name(w12261) -> ("单组电压不均衡"=w12260:dbl)
                    n4699 = call "输入分辨率计算-EV05.vi"("1字节?"=FALSE, "数值"=w12260, "偏移量"=0.0, "分辨率"=0.001) -> ("低字节"=w12262:dbl, "高字节1"=w12264:dbl)  [unwired: 1 in, 5 out]
                  }
                  frame Enabled {
                    w12267 = 255 ("高字节1")
                  }
                }
                n4700 = Build Array(w12259, w12257) -> (w12258:i32[])
              }
              frame 6 {
                # "整组电压不均衡"
                n4701 = disable-structure shown="启用" {
                  disable-tunnel: [w12276 w12279] -> w12271
                  disable-tunnel: [w12274 w12279] -> w12269
                  disable-tunnel: w12268 -> [w12273 _]
                  frame Disabled {
                    n4702 = Unbundle By Name(w12273) -> ("整组电压不均衡"=w12272:dbl)
                    n4703 = call "输入分辨率计算-EV05.vi"("1字节?"=FALSE, "数值"=w12272, "偏移量"=0.0, "分辨率"=0.001) -> ("低字节"=w12274:dbl, "高字节1"=w12276:dbl)  [unwired: 1 in, 5 out]
                  }
                  frame Enabled {
                    w12279 = 255 ("高字节1")
                  }
                }
                n4704 = Build Array(w12271, w12269) -> (w12270:i32[])
              }
              frame 7 {
                # "单体电压过高"
                n4705 = disable-structure shown="启用" {
                  disable-tunnel: [w12288 w12291] -> w12283
                  disable-tunnel: [w12286 w12291] -> w12281
                  disable-tunnel: w12280 -> [w12285 _]
                  frame Disabled {
                    n4706 = Unbundle By Name(w12285) -> ("单体电压过高"=w12284:dbl)
                    n4707 = call "输入分辨率计算-EV05.vi"("1字节?"=FALSE, "数值"=w12284, "偏移量"=0.0, "分辨率"=0.001) -> ("低字节"=w12286:dbl, "高字节1"=w12288:dbl)  [unwired: 1 in, 5 out]
                  }
                  frame Enabled {
                    w12291 = 255 ("高字节1")
                  }
                }
                n4708 = Build Array(w12283, w12281) -> (w12282:i32[])
              }
              frame 8 {
                # "单体电压过低"
                n4709 = disable-structure shown="启用" {
                  disable-tunnel: [w12300 w12303] -> w12295
                  disable-tunnel: [w12298 w12303] -> w12293
                  disable-tunnel: w12292 -> [w12297 _]
                  frame Disabled {
                    n4710 = Unbundle By Name(w12297) -> ("单体电压过低"=w12296:dbl)
                    n4711 = call "输入分辨率计算-EV05.vi"("1字节?"=FALSE, "数值"=w12296, "偏移量"=0.0, "分辨率"=0.001) -> ("低字节"=w12298:dbl, "高字节1"=w12300:dbl)  [unwired: 1 in, 5 out]
                  }
                  frame Enabled {
                    w12303 = 255 ("高字节1")
                  }
                }
                n4712 = Build Array(w12295, w12293) -> (w12294:i32[])
              }
              frame 9 {
                # "充电电流过高"
                n4713 = disable-structure shown="启用" {
                  disable-tunnel: [w12312 w12315] -> w12307
                  disable-tunnel: [w12310 w12315] -> w12305
                  disable-tunnel: w12304 -> [w12309 _]
                  frame Disabled {
                    n4714 = Unbundle By Name(w12309) -> ("充电电流过高"=w12308:dbl)
                    n4715 = call "输入分辨率计算-EV05.vi"("1字节?"=FALSE, "数值"=w12308, "偏移量"=-3000.0, "分辨率"=0.1) -> ("低字节"=w12310:dbl, "高字节1"=w12312:dbl)  [unwired: 1 in, 5 out]
                  }
                  frame Enabled {
                    w12315 = 255 ("高字节1")
                  }
                }
                n4716 = Build Array(w12307, w12305) -> (w12306:i32[])
              }
              frame 10 {
                # "放电电流过高"
                n4717 = disable-structure shown="启用" {
                  disable-tunnel: [w12324 w12327] -> w12319
                  disable-tunnel: [w12322 w12327] -> w12317
                  disable-tunnel: w12316 -> [w12321 _]
                  frame Disabled {
                    n4718 = Unbundle By Name(w12321) -> ("放电电流过高"=w12320:dbl)
                    n4719 = call "输入分辨率计算-EV05.vi"("1字节?"=FALSE, "数值"=w12320, "偏移量"=-3000.0, "分辨率"=0.1) -> ("低字节"=w12322:dbl, "高字节1"=w12324:dbl)  [unwired: 1 in, 5 out]
                  }
                  frame Enabled {
                    w12327 = 255 ("高字节1")
                  }
                }
                n4720 = Build Array(w12319, w12317) -> (w12318:i32[])
              }
              frame 11 {
                # "单组温度不均衡"
                n4721 = disable-structure shown="启用" {
                  disable-tunnel: [w12334 255 ("高字节1")] -> w12330
                  disable-tunnel: w12328 -> [w12332 _]
                  frame Disabled {
                    n4722 = Unbundle By Name(w12332) -> ("单组温度不均衡"=w12331:dbl)
                    n4723 = call "输入分辨率计算-EV05.vi"("1字节?"=TRUE, "数值"=w12331, "偏移量"=0.0, "分辨率"=1.0) -> ("高字节1"=w12334:dbl)  [unwired: 1 in, 6 out]
                  }
                  frame Enabled {
                  }
                }
                n4724 = Build Array(w12330) -> (w12329:i32[])
              }
              frame 12 {
                # "SOC过高"
                n4725 = Unbundle By Name(w12340) -> ("SOC过高"=w12339:dbl)
                n4726 = call "输入分辨率计算-EV05.vi"("1字节?"=FALSE, "数值"=w12339, "偏移量"=0.0, "分辨率"=0.1) -> ()  [unwired: 1 in, 7 out]
                n4727 = disable-structure shown="启用" {
                  disable-tunnel: _ -> [w12346 _]
                  disable-tunnel: [w12346 255 ("高字节1")] -> w12338
                  disable-tunnel: [w12345 i32[] [] ("低位子数组")] -> _
                  disable-tunnel: _ -> [w12345 _]
                  frame Disabled {
                  }
                  frame Enabled {
                  }
                }
                n4728 = Build Array(w12338, w12338) -> (w12342:i32[])
              }
              frame 13 {
                # "SOC过低"
                n4729 = Unbundle By Name(w12352) -> ("SOC过低"=w12351:dbl)
                n4730 = call "输入分辨率计算-EV05.vi"("1字节?"=FALSE, "数值"=w12351, "偏移量"=0.0, "分辨率"=0.1) -> ("低字节"=w12349:dbl, "高字节1"=w12350:dbl)  [unwired: 1 in, 5 out]
                n4731 = Build Array(w12350, w12349) -> (w12354:dbl[])
              }
              frame 14 {
                # "内阻过大"
                n4732 = disable-structure shown="启用" {
                  disable-tunnel: w12359 -> [w12364 _]
                  disable-tunnel: [w12360 255 ("高字节1")] -> w12357
                  frame Disabled {
                    n4733 = Unbundle By Name(w12364) -> ("内阻过大"=w12363:dbl)
                    n4734 = call "输入分辨率计算-EV05.vi"("1字节?"=TRUE, "数值"=w12363, "分辨率"=0.1) -> ("高字节1"=w12360:dbl)  [unwired: 2 in, 6 out]
                  }
                  frame Enabled {
                  }
                }
                n4735 = Build Array(w12357) -> (w12358:i32[])
              }
              frame 15 {
                # "极柱温度过高"
                n4736 = disable-structure shown="启用" {
                  disable-tunnel: w12368 -> [w12374 _]
                  disable-tunnel: [w12370 255 ("高字节1")] -> w12366
                  frame Disabled {
                    n4737 = Unbundle By Name(w12374) -> ("极柱温度过高"=w12373:dbl)
                    n4738 = call "输入分辨率计算-EV05.vi"("1字节?"=TRUE, "数值"=w12373, "偏移量"=-40.0, "分辨率"=1.0) -> ("高字节1"=w12370:dbl)  [unwired: 1 in, 6 out]
                  }
                  frame Enabled {
                  }
                }
                n4739 = Build Array(w12366) -> (w12367:i32[])
              }
              frame 16 {
                # "SOH过低"
                n4740 = disable-structure shown="启用" {
                  disable-tunnel: [w12391 w12399] -> w12378
                  disable-tunnel: w12377 -> [w12388 _]
                  disable-tunnel: [w12380 w12399] -> w12376
                  frame Disabled {
                    n4741 = Unbundle By Name(w12388) -> ("SOH过低"=w12387:dbl)
                    n4742 = call "输入分辨率计算-EV05.vi"("1字节?"=FALSE, "数值"=w12387, "偏移量"=0.0, "分辨率"=0.1) -> ("低字节"=w12389:dbl, "高字节1"=w12390:dbl)  [unwired: 1 in, 5 out]
                    n4743 = call "二进制解析-8.6.vi"("索引"=4, "数值"=w12390) -> ("低位子数组"=w12393:i32[])  [unwired: 3 out]
                    n4744 = call "二进制解析-8.6.vi"("索引"=4, "数值"=w12389) -> ("低位子数组"=w12382:i32[], "高位子数组"=w12392:i32[])  [unwired: 2 out]
                    n4745 = call "二进制解析-8.6.vi"("索引"=4, "数值"=0) -> ("低位子数组"=w12383:i32[])  [unwired: 3 out]
                    n4746 = Insert Into Array(array=w12393, new element=w12392) -> (w12386:i32[])  [unwired: 1 in]
                    n4747 = Insert Into Array(array=w12382, new element=w12383) -> (w12381:i32[])  [unwired: 1 in]
                    n4748 = call "数值二进制转十进制-8.6.vi"("子数组"=w12386) -> ("十进制数值"=w12391:i32)  [unwired: 4 out]
                    n4749 = call "数值二进制转十进制-8.6.vi"("子数组"=w12381) -> ("十进制数值"=w12380:i32)  [unwired: 4 out]
                  }
                  frame Enabled {
                    w12399 = 255 ("高字节1")
                  }
                }
                n4750 = Build Array(w12378, w12376) -> (w12379:i32[])
              }
            }
            n4751 = Insert Into Array(array=w12200, new element=w12201) -> (w12199:dbl[])  [unwired: 1 in]
          }
